vi "Average.vi"(11 "p_atm":sgl) -> (3 "Average value":sgl)   [LabVIEW 2020]
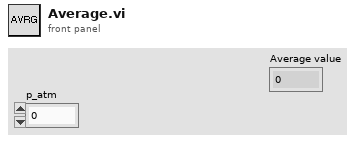
[diagram p1: front panel]
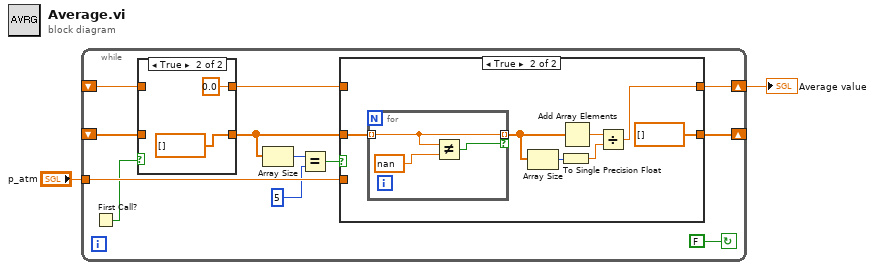
[diagram p0: block diagram]
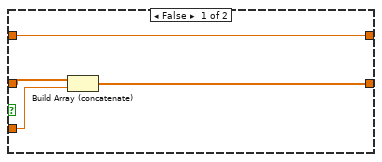
[diagram p3: hidden frame]
diagram:
  n1 = while {
    tunnel: "p_atm" -> [w14]
    shift-right: [w11] -> _
    shift-left: _ -> [w6]
    shift-right: [w13] -> w1
    shift-left: _ -> [w4]
    stop <- FALSE continue-if-true
    n2 = First Call?() -> (First Call?: T/F=w7:bool)
    n3 = case shown="True" w7 {
      tunnel: w6 -> [w16 _]
      tunnel: [w16 sgl[] []] -> w5
      tunnel: w4 -> [w15 _]
      tunnel: [w15 sgl 0.0] -> w3
      frame False {
      }
      frame True {
      }
    }
    n4 = Array Size(array=w5) -> (size(s)=w10:i32)
    n5 = Equal?(x=w10, y=5) -> (x = y?=w8:bool)
    n6 = case shown="True" w8 {
      tunnel: w14 -> [w22 _]
      tunnel: [w19 w25] -> w13
      tunnel: [w20 sgl[] []] -> w11
      tunnel: w5 -> [w21 w28]
      tunnel: w3 -> [w19 _]
      frame False {
        n7 = Build Array (concatenate)(w21, w22) -> (w20:sgl[])
      }
      frame True {
        n8 = for {
          tunnel: w28 -> [w32] mode=indexing
          tunnel: [w32] -> w23 mode=indexing if=w31
          n9 = Not Equal?(x=w32, y=sgl nan) -> (x != y?=w31:bool)
        }
        n10 = Array Size(array=w23) -> (size(s)=w27:i32)
        n11 = To Single Precision Float(number=w27) -> (single precision float=w26:sgl)
        n12 = Add Array Elements(numeric array=w23) -> (sum=w24:sgl)
        n13 = Divide(x=w24, y=w26) -> (x/y=w25:sgl)
      }
    }
  }
  "Average value" <- w1
